vi "testConverDatatype.vi"(11 "queuein":string) -> (3 "queueout":string)   [LabVIEW 2011]
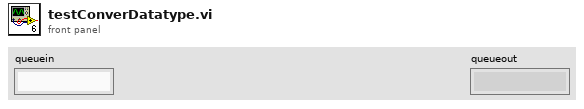
[diagram p1: front panel]
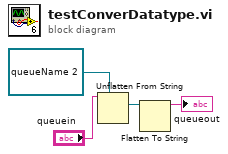
[diagram p0: block diagram]
diagram:
  n1 = Unflatten From String(type=refnum<queue> refnum ("队列输出"), binary string="queuein") -> (value=w2:refnum<queue>)  [unwired: 3 in, 2 out]
  n2 = Flatten To String(anything=w2) -> (data string=→"queueout":string)  [unwired: 3 in, 2 out]
